vi "set plot style.vi"(8 "error in (no error)":errorcluster, 9 "single point style":i32=2, 10 "streak length":i32, 11 "XYGraph in":refnum<vi>) -> (0 "error out":errorcluster)   [LabVIEW 2020]
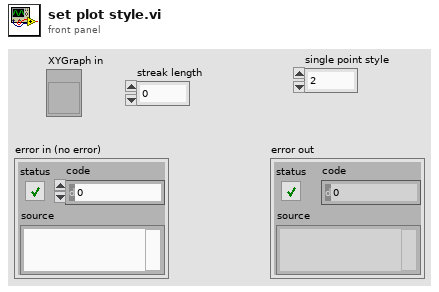
[diagram p1: front panel]
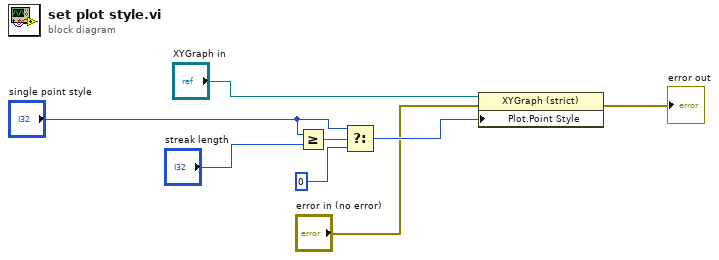
[diagram p0: block diagram]
diagram:
  n1 = Greater Or Equal?(x="single point style", y="streak length") -> (x >= y?=w7:bool)
  n2 = Select(t="single point style", s=w7, f=0) -> (s? t:f=w3:i32)
  n3 = property class="XYGraph (strict)"(reference="XYGraph in", error in="error in (no error)", "Plot.Point Style"=w3) -> (error out=→"error out":errorcluster)  [unwired: 1 out]
